vi "Set Delay After Transaction.vi"(8 "error in (no error)":errorcluster, 10 "delay, ms":u32, 11 "MODBUS in":refnum<class "PL Modbus Client.lvclass">) -> (0 "error out":errorcluster, 3 "MODBUS out":refnum<class "PL Modbus Client.lvclass">)   [LabVIEW 2015, in "PL Modbus Client.lvclass"]
doc: "Sets delay after transaction. This can be useful when RS-485 device is slow to release the interface."
uses:
  PL Modbus Client.lvclass
  PL Modbus Client.lvclass/PL Modbus Client.ctl
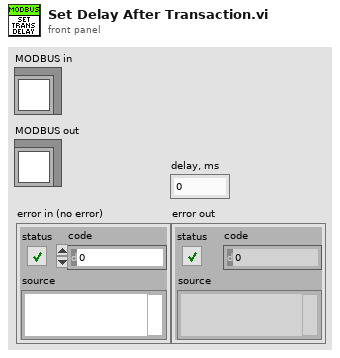
[diagram p1: front panel]
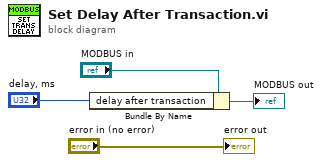
[diagram p0: block diagram]
diagram:
  n1 = Bundle By Name(cluster="MODBUS in", "delay after transaction"="delay, ms") -> (→"MODBUS out":refnum<class "PL Modbus Client.lvclass">)
  "error out" <- "error in (no error)"
